vi "To Pythonic - Float.vi"(3 "Precision (6)":i16, 4 "Float":dbl) -> (1 "Pythonic Value":string)   [LabVIEW 2012, in "OPI.lvclass"]
doc: "Convert LabVIEW data into valid pythonic representation."
uses:
  OPI.lvclass
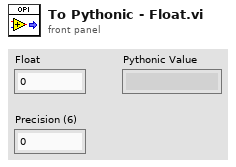
[diagram p1: front panel]
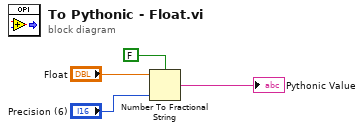
[diagram p0: block diagram]
diagram:
  n1 = Number To Fractional String(use system decimal point (T)=FALSE, number="Float", precision (6)="Precision (6)") -> (F-format string=→"Pythonic Value":string)  [unwired: 1 in]
